vi "Snippets.vi"(6 "args":string[](array[string]), 7 "QD Plugins Dir":path, 8 "error in (no error)":errorcluster, 9 "Shift?":bool, 10 "Focus":enum8{"FP", "BD"}(ring), 11 "VI Refnum":refnum<vi>) -> (0 "error out":errorcluster)   [LabVIEW 2019]
doc: "Imports or exports a VI Snippet (*.png) image programmatically. Import opens a preview dialog to select a VI Snippet (*.png) from the <b>QuickDrop\\plugins\\Snippets</b> directory. Export prompts the user where to save the VI Snippet (*.png). On export, if nothing is selected the entire VI is exported. Otherwise only the selected Block Diagram GObjects are exported.\n\n[SCRIPT]\nimport=Import VI Snippet\nexport=Export VI Snippet"
uses:
  _Snippets/VI Snippet.lvlibp/1abvi3w/vi.lib/Utility/miscctls.llb/LVPositionTypeDef.ctl
  _Snippets/VI Snippet.lvlibp
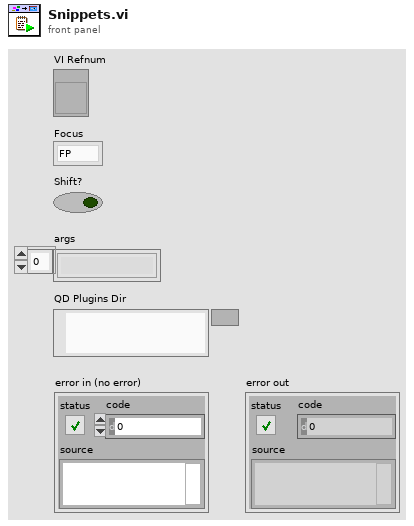
[diagram p1: front panel]
types:
  T1 = typedef "VI Snippet.lvlibp/LVPositionTypeDef.ctl" = cluster{"Left":i32, "Top":i32}
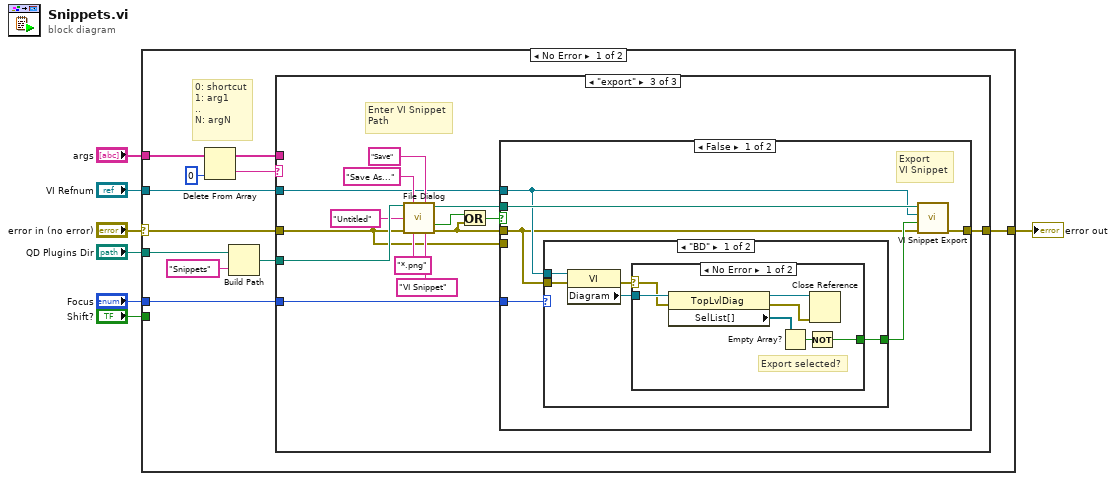
[diagram p0: block diagram]
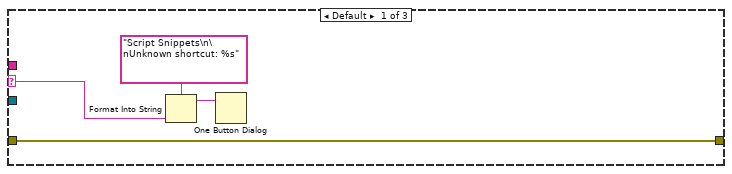
[diagram p2: hidden frame]
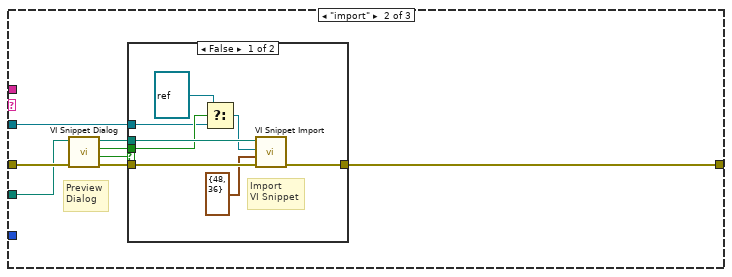
[diagram p3: hidden frame]
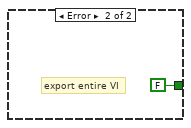
[diagram p5: hidden frame]
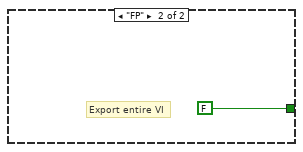
[diagram p6: hidden frame]
diagram:
  n1 = case shown="No Error" "error in (no error)" {
    selector: "error in (no error)" -> [w14 w75]
    tunnel: "VI Refnum" -> [w9 _]
    tunnel: "Focus" -> [w8 _]
    tunnel: "Shift?" -> [_ _]
    tunnel: "args" -> [w17 _]
    tunnel: [w13 w75] -> w2
    tunnel: "QD Plugins Dir" -> [w11 _]
    frame No Error {
      # "0: shortcut\n1: arg1\n..\nN: argN"
      n2 = Delete From Array(array=w17, index=0) -> (deleted portion=w16:string, array with subset deleted=w15:string[])  [unwired: 1 in]
      n3 = Build Path(base path=w11, name or relative path="Snippets") -> (appended path=w12:path)
      n4 = case shown="\"export\"" w16 {
        selector: w16 -> [w19 _ _]
        tunnel: [w22 w27 w45] -> w13
        tunnel: w14 -> [w22 w30 w46]
        tunnel: w15 -> [_ _ _]
        tunnel: w12 -> [_ w29 w53]
        tunnel: w9 -> [_ w24 w42]
        tunnel: w8 -> [_ _ w41]
        frame Default {
          n5 = Format Into String(format string="Script Snippets\n\nUnknown shortcut: %s", w19) -> (resulting string=w20:string)  [unwired: 2 in, 1 out]
          n6 = One Button Dialog(message=w20) -> ()  [unwired: 1 in, 1 out]
        }
        frame "import" {
          # "Preview\nDialog"
          n7 = call "VI Snippet Dialog.vi"("error in (no error)"=w30, "VI Snippets Dir"=w29) -> ("error out"=w28:errorcluster, "Cancelled?"=w23:bool, "New VI?"=w25:bool, "VI Snippets Path"=w26:path)  [unwired: 6 in]
          n8 = case shown="False" w23 {
            tunnel: w28 -> [w38 w39]
            tunnel: [w37 w39] -> w27
            tunnel: w26 -> [w36 _]
            tunnel: w25 -> [w35 _]
            tunnel: w24 -> [w33 _]
            frame False {
              # "Import\nVI Snippet"
              n9 = Select(t=refnum<vi> refnum, s=w35, f=w33) -> (s? t:f=w34:refnum<vi>)
              n10 = call "VI Snippet Import.vi"("error in (no error)"=w38, "Drop Position (0, 0)"=T1 {"Left"=48, "Top"=36}, "VI Refnum in (NaN=New VI)"=w34, "VI Snippet Path (*.png)"=w36) -> ("error out"=w37:errorcluster)  [unwired: 4 in, 3 out]
            }
            frame True {
              # "Cancelled"
            }
          }
        }
        frame "export" {
          # "Enter VI Snippet\nPath"
          n11 = call "File Dialog"("start path"=w53, "prompt"="Save As...", "button label"="Save", "default name"="Untitled", "error in"=w46, "pattern (all files)"="*.png", "pattern label"="VI Snippet") -> ("selected path"=w44:path, "cancelled"=w48:bool, "error out"=w43:errorcluster)  [unwired: 5 in, 1 out]
          n12 = Or(x=w48, y=w43) -> (x .or. y?=w47:bool)
          n13 = case shown="False" w47 {
            tunnel: w46 -> [_ w74]
            tunnel: [w58 w74] -> w45
            tunnel: w44 -> [w59 _]
            tunnel: w43 -> [w54 _]
            tunnel: w42 -> [w55 _]
            tunnel: w41 -> [w56 _]
            frame False {
              # "Export\nVI Snippet"
              n14 = case shown="\"BD\"" w56 {
                tunnel: [w61 FALSE ("Selected GObjects Only? (F)")] -> w57
                tunnel: w55 -> [w64 _]
                tunnel: w54 -> [w60 _]
                frame "BD" {
                  n15 = property class="VI"(reference=w64, error in=w60) -> (error out=w62:errorcluster, "Diagram"=w63:refnum<vi>)  [unwired: 1 out]
                  n16 = case shown="No Error" w62 {
                    selector: w62 -> [w70 _]
                    tunnel: w63 -> [w71 _]
                    tunnel: [w65 FALSE] -> w61
                    frame No Error {
                      # "Export selected?"
                      n17 = property class="TopLvlDiag"(reference=w71, error in=w70) -> (reference out=w68:refnum<vi>, error out=w67:errorcluster, "SelList[]"=w69:refnum<vi>[])
                      n18 = Empty Array?(array=w69) -> (empty?=w66:bool)
                      n19 = Not(x=w66) -> (.not. x?=w65:bool)
                      n20 = Close Reference(reference=w68, error in (no error)=w67) -> ()  [unwired: 1 out]
                    }
                    frame Error {
                      # "export entire VI"
                    }
                  }
                }
                frame "FP" {
                  # "Export entire VI"
                }
              }
              n21 = call "VI Snippet Export.vi"("error in (no error)"=w54, "Selected GObjects Only? (F)"=w57, "VI Refnum"=w55, "VI Snippet Path (*.png)"=w59) -> ("error out"=w58:errorcluster)  [unwired: 7 in]
            }
            frame True {
              # "Cancelled"
            }
          }
        }
      }
    }
    frame Error {
    }
  }
  "error out" <- w2
